vi "forceOutputState.vi"(8 "error in (no error)":errorcluster, 9 "calibratedValues":dbl[](array[numeric]), 10 "channel_addresses":string[](array[string]), 11 "DIO64Output in":refnum<class "DIO64Output.lvclass">) -> (0 "error out":errorcluster, 3 "DIO64Output out":refnum<class "DIO64Output.lvclass">)   [LabVIEW 2009, in "Hardware.lvlib" / "Channels.lvlib" / "DIO64Output.lvclass"]
uses:
  DIO64Output.lvclass
  <userlib>/dio64_32.LLB/DIO64 Out Config Control.ctl
  <userlib>/dio64_32.LLB/DIO64 clock control.ctl
  <userlib>/dio64_32.LLB/DIO64 start trig.ctl
  <userlib>/dio64_32.LLB/DIO64 stop trig.ctl
  DIO64Output.lvclass/DIO64Output.ctl
  DigitalOutput.lvclass
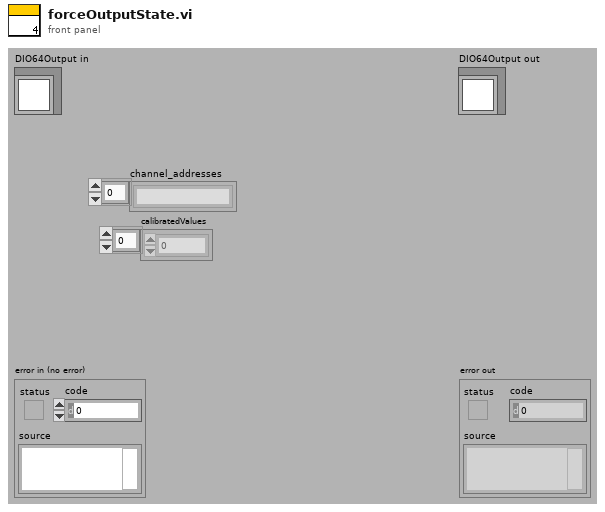
[diagram p1: front panel]
types:
  T1 = typedef "DIO64 Out Config Control.ctl" = cluster{"flags":enum16{"unused"}, "clock control":T2, "start trigger":T3, "stop trigger":T4, "DAQ clock modulo":u32, "repetitions":u32, "#transitions":u16}
  T2 = typedef "DIO64 clock control.ctl" = enum16{"internal", "external", "trig 0", "OCXO"}
  T3 = typedef "DIO64 start trig.ctl" = cluster{"source":enum16{"none", "internal", "external", "trig 2", "PXI Star"}, "type":enum16{"level", "edge", "edge to edge"}, "sense":enum16{"rising", "falling"}}
  T4 = typedef "DIO64 stop trig.ctl" = cluster{"source":enum16{"none", "internal", "external", "trig 3 in", "output FIFO"}, "type":enum16{"level", "edge"}, "sense":enum16{"falling", "rising"}}
  T5 = cluster{"channel_addresses":string[], "calibratedValues":dbl[]}
  T6 = typedef "DIO64 Out Status.ctl" = cluster{"pktsize":u16, "portCount":u16, "writePtr":u16, "readPtr":u16, "time0":u16, "time1":u16, "fifoSize":u32, "fifo0":u16, "ticks":u32, "flags":u16, "clkControl":u16, "startControl":u16, "stopControl":u16, "AIControl":u32, "AICurrent":u16, "startTime0":u16, "startTime1":u16, "stopTime0":u16, "stopTime1":u16, "cur trans":u32, "cur reps":u32}
  T7 = cluster{"Timestamps ms":dbl[], "DataPerChannel":dbl[][]}
  T8 = cluster{"Timestamps ms":dbl[], "Bitmap":bool[][]}
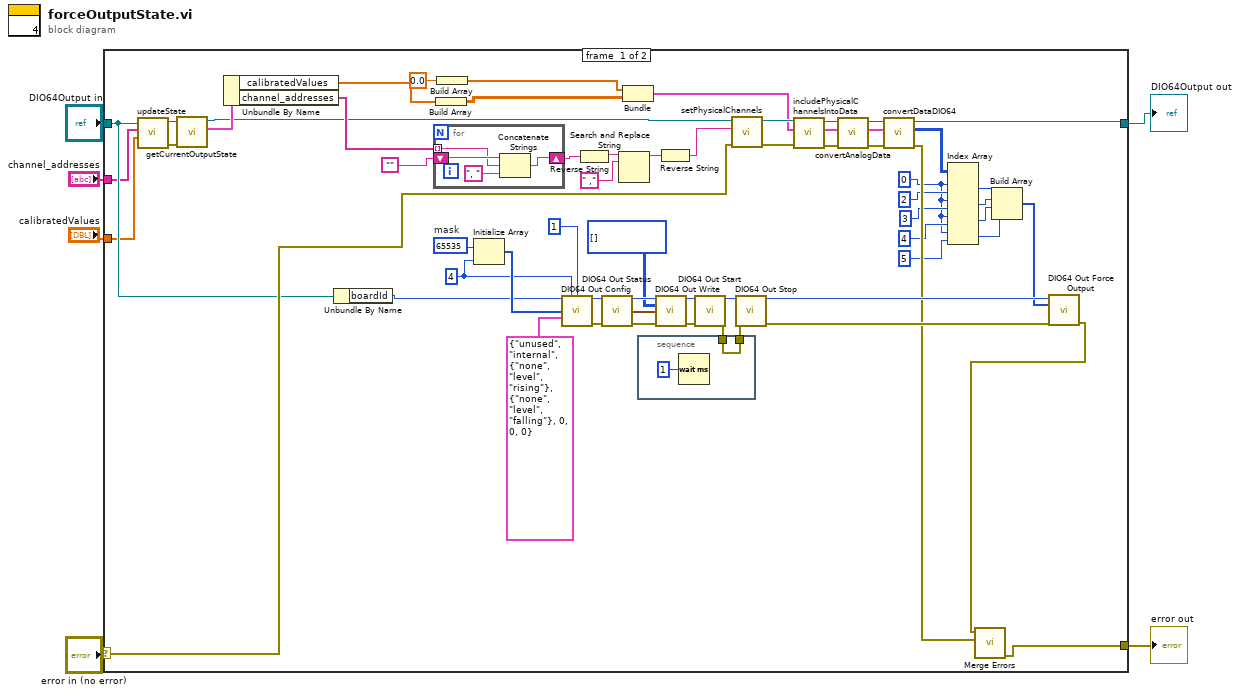
[diagram p0: block diagram]
diagram:
  n1 = case shown="No Error" "error in (no error)" {
    selector: "error in (no error)" -> [w26 w75]
    tunnel: [w29 w76] -> w5
    tunnel: "DIO64Output in" -> [w15 w76]
    tunnel: [w28 w75] -> w3
    tunnel: "calibratedValues" -> [w13 _]
    tunnel: "channel_addresses" -> [w14 _]
    frame #0 {
      w58 = u16 65535  # mask
      w22 = 0
      w59 = 4
      n2 = call "updateState.vi"("calibratedValues"=w13, "channel_addresses"=w14, "DigitalOutput in"=w15) -> ("error out"=w11:errorcluster, "DigitalOutput out"=w12:refnum<class "DIO64Output.lvclass">)  [unwired: 7 in]
      n3 = call "getCurrentOutputState.vi"("error in (no error)"=w11, "DigitalOutput.lvclass in"=w12) -> ("CurrentOutputState"=w10:T5, "DigitalOutput.lvclass out"=w7:refnum<class "DIO64Output.lvclass">)  [unwired: 7 in, 1 out]
      n4 = Unbundle By Name(w10) -> ("calibratedValues"=w9:dbl[], "channel_addresses"=w8:string[])
      n5 = Unbundle By Name(w15) -> ("boardId"=w30:i32)
      n6 = for {
        shift-right: [w70] -> w47
        shift-left: "" -> [w72]
        tunnel: w8 -> [w69] mode=indexing
        n7 = Concatenate Strings(w72, w69, ", ") -> (w70:string)
      }
      n8 = Build Array(w9) -> (w39:dbl[][])
      n9 = Build Array(0.0) -> (w40:dbl[])
      n10 = Initialize Array(w58, w59) -> (w60:u16[])
      n11 = call <userlib>:"DIO64 Out Config.vi"("board in"=w30, "#ports"=w59, "divider"=u32 1, "mask"=w60, "Config Control"=T1 {"flags"=enum."unused", "clock control"=enum."internal", "start trigger"={"source"=enum."none", "type"=enum."level", "sense"=enum."rising"}, "stop trigger"={"source"=enum."none", "type"=enum."level", "sense"=enum."falling"}, "DAQ clock modulo"=0, "repetitions"=0, "#transitions"=0}) -> ("board out"=w67:u16, "error out"=w68:errorcluster)  [unwired: 8 in, 1 out]
      n12 = Reverse String(1:w47) -> (0:w46:string)
      n13 = call <userlib>:"DIO64 Out Status.vi"("board in"=w67, "error in (no error)"=w68) -> ("board out"=w64:u16, "Out Status"=w63:T6, "error out"=w61:errorcluster)  [unwired: 10 in, 1 out]
      n14 = Search and Replace String(input string=w46, search string=" ,") -> (result string=w44:string)  [unwired: 6 in, 3 out]
      n15 = Bundle(w40, w39) -> (w27:cluster{dbl[], dbl[][]})  [unwired: 1 in]
      n16 = call <userlib>:"DIO64 Out Write.vi"("board in"=w64, "data"=u16[][] [] ("Timestamp and Data Array for each board"), "Out Status"=w63, "error in (no error)"=w61) -> ("board out"=w65:u16, "error out"=w62:errorcluster)  [unwired: 10 in]
      n17 = Reverse String(1:w44) -> (0:w43:string)
      n18 = call <userlib>:"DIO64 Out Start.vi"("board in"=w65, "error in (no error)"=w62) -> ("board out"=w66:u16, "error out"=w55:errorcluster)  [unwired: 12 in]
      n19 = stacked-sequence {
        tunnel: w55 -> [w74]
        tunnel: [w74] -> w54
        frame #0 {
          n20 = Wait (ms)(milliseconds to wait=u32 1) -> ()  [unwired: 1 out]
        }
      }
      n21 = call-dynamic "setPhysicalChannels.vi"("error in (no error)"=w26, "Physical Channels"=w43, "DigitalOutput.lvclass in"=w7) -> ("error out"=w41:errorcluster, "DigitalOutput.lvclass out"=w42:refnum<class "DIO64Output.lvclass">)  [unwired: 7 in]
      n22 = call <userlib>:"DIO64 Out Stop.vi"("board in"=w66, "error in (no error)"=w54) -> ("board out"=w51:u16, "error out"=w52:errorcluster)  [unwired: 12 in]
      n23 = call "includePhysicalChannelsIntoData.vi"("error in (no error)"=w41, "Data"=w27, "DIO64Output in"=w42) -> ("error out"=w38:errorcluster, "Data out"=w36:T7, "DIO64Output out"=w37:refnum<class "DIO64Output.lvclass">)  [unwired: 6 in]
      n24 = call "convertAnalogData.vi"("error in (no error)"=w38, "Data"=w36, "DIO64Output in"=w37) -> ("error out"=w34:errorcluster, "digitalData"=w35:T8, "DIO64Output out"=w33:refnum<class "DIO64Output.lvclass">)  [unwired: 6 in]
      n25 = call "convertDataDIO64.vi"("error in (no error)"=w34, "Data"=w35, "DIO64Output in"=w33) -> ("error out"=w31:errorcluster, "data"=w32:u16[][], "DIO64Output out"=w29:refnum<class "DIO64Output.lvclass">)  [unwired: 4 in, 2 out]
      n26 = Index Array(array=w32, index (row) #1=w22, index (col) #1=2, index (row) #2=w22, index (col) #2=3, index (row) #3=w22, index (col) #3=4, index (row) #4=w22, index (col) #4=5) -> (element #1=w20:u16, element #2=w19:u16, element #3=w18:u16, element #4=w17:u16)
      n27 = Build Array(w20, w19, w18, w17) -> (w16:u16[])
      n28 = call <userlib>:"DIO64 Out Force Output.vi"("board in"=w51, "data"=w16, "error in (no error)"=w52) -> ("error out"=w50:errorcluster)  [unwired: 11 in, 1 out]
      n29 = call <vilib>:"Merge Errors.vi"("error in 2 (no error)"=w31, "error in 1 (no error)"=w50) -> ("error out"=w28:errorcluster)  [unwired: 5 in]
    }
    frame #1 {
    }
  }
  "error out" <- w3
  "DIO64Output out" <- w5
